vi "PNA_yokogawa_anritsu_combined.vi"() -> ()   [LabVIEW 2020]
uses:
  <vilib>/Utility/file.llb/Write Delimited Spreadsheet (DBL).vi
  <instrlib>/Keysight PNA Series/Keysight PNA Series.lvlib
  <instrlib>/Anritsu MG369X Series/Anritsu MG369X Series.lvlib
  <instrlib>/Yokogawa 7651/Yokogawa 7651.lvlib
panel:
  in  "Increment cluster":T1={"Yoko_Increment"=0.02, "Micro_Increment (GHz)"=0.1}
  in  "PNA_control":T2={"Channel (1)"=1, "Start Frequency (Hz)"=1000000.0, "Stop Frequency (Hz)"=10000000000.0, "Sweep Points (201)"=201, "Sweep Type (0: Linear)"=0, "Sweep Generation (1: Analog)"=1, "Bandwidth (Hz)"=100000.0, "Average Count (1)"=1, "Enable Average "=FALSE, "Power"={"Attenuation (0 dB)"=0.0, "Power Level (0 dBm)"=0.0, "Enable Auto Attenuation"=TRUE, "Enable RF Power"=TRUE, "Enable Power Slope"=FALSE, "Port (1)"=1, "Power Slope (0 dB/GHz)"=0.0}, "Enable Reduce IF Bandwidth "=TRUE, "Electrical delay"={"Unit (0: Meter)"=0, "Waveguide Cutoff Frequency (Hz)"=45000000.0, "Distance (0)"=0.0, "Medium "=0, "Delay (0 s)"=0.0}, "Measurement name"=[], "Measurement Parameters (S11)"=[]} {"Electrical delay"."Medium" items=["Coaxial", "Waveguide"]; "Electrical delay"."Unit (0: Meter)" items=["Meter", "Feet", "Inch"]; "Sweep Generation (1: Analog)" items=["Stepped", "Analog"]; "Sweep Type (0: Linear)" items=["Linear", "Logarithmic", "Power", "CW", "Segment", "Phase"]}
  in  "VNA_force_stop":bool
  in  "Save?":bool
  in  "Save file path":path=path "D:/Sheng-Xiang_Lin/JPA"
  in  "File_name":string="JPA"
  in  "Yoko_control":T3={"Range"=enum."10mA", "Init_Current/ Voltage "=1.46}
  in  "Output_control":T4
  in  "MicroScan_or_YokoScan":enum16{"MicroScan", "YokoScan"}(ring)=enum."YokoScan"
  in  "Display format 1-2":T5={"Display Format 2"=3, "Display Format 1"=1} {"Display Format 1" items=["Magnitude Linear", "Magnitude Logarithmic", "Phase", "Unwrapped phase", "Imaginary", "Real", "Polar", "Smith Chart", "Smith Admittance", "SWR", "Group Delay", "Kelvin", "Fahrenheit", "Celsius"]; "Display Format 2" items=["Magnitude Linear", "Magnitude Logarithmic", "Phase", "Unwrapped phase", "Imaginary", "Real", "Polar", "Smith Chart", "Smith Admittance", "SWR", "Group Delay", "Kelvin", "Fahrenheit", "Celsius"]}
  out "average_times":i32=1
  in  "MG369X_control":T6={"Initial Frequency (Hz)"=4000000000.0, "Initial Power Level (dBm)"=0.0, "Trigger Type (1: Free Run)"=1, "Clock Rate (4: Clock 100)"=1, "Trigger Edge Type (0: Trigger Rising)"=0, "Polarity (1: High RF On)"=1, "Pulse_Period (s)"=1e-08, "Mode (1: Single)"=1, "Reset (True)"=FALSE, "ID Query (True)"=FALSE} {"Mode (1: Single)" items=["Single"=1, "Doublet"=2, "Triplet"=3, "Quadruplet"=4]; "Pulse_Period (s)" format="%#_12g"; "Polarity (1: High RF On)" items=["Low RF On", "High RF On"]; "Trigger Edge Type (0: Trigger Rising)" items=["Trigger Rising", "Trigger Falling"]; "Clock Rate (4: Clock 100)" items=["Clock 10"=1, "Clock 100"=4]; "Trigger Type (1: Free Run)" items=["Free Run"=1, "Gated"=2, "Delayed"=3, "Triggered"=4, "Triggered w/delay"=5]}
  in  "Force_stop":bool
  out "State":T7(ring)=enum."Close"
  in  "Limit_Cluster":T8={"Current_or_voltage_limit"=1.5, "Micro_freq_limit (GHz)"=4.5}
  in  "Current_Value":T9={"Yoko_Current_or_Voltage"=1.52, "Micro_frequency (GHz)"=4.0, "Ch1 Intensity Graph"=array2001x3[6003 elements], "Freq_Array"=array[2001 elements], "Ch2 Intensity Graph"=array2001x3[6003 elements], "Ch1"={"Magnitude"=array[201 elements], "Phase"=array[201 elements]}, "Ch2"={"Magnitude"=array[201 elements], "Phase"=array[201 elements]}}
  in  "Leave_pend":bool
  in  "Visa_Cluster":T10={"VNA visa"="GPIB0::16::INSTR", "MG369x visa"="GPIB0::5::INSTR", "Yokogawa visa"="GPIB0::1::INSTR"}
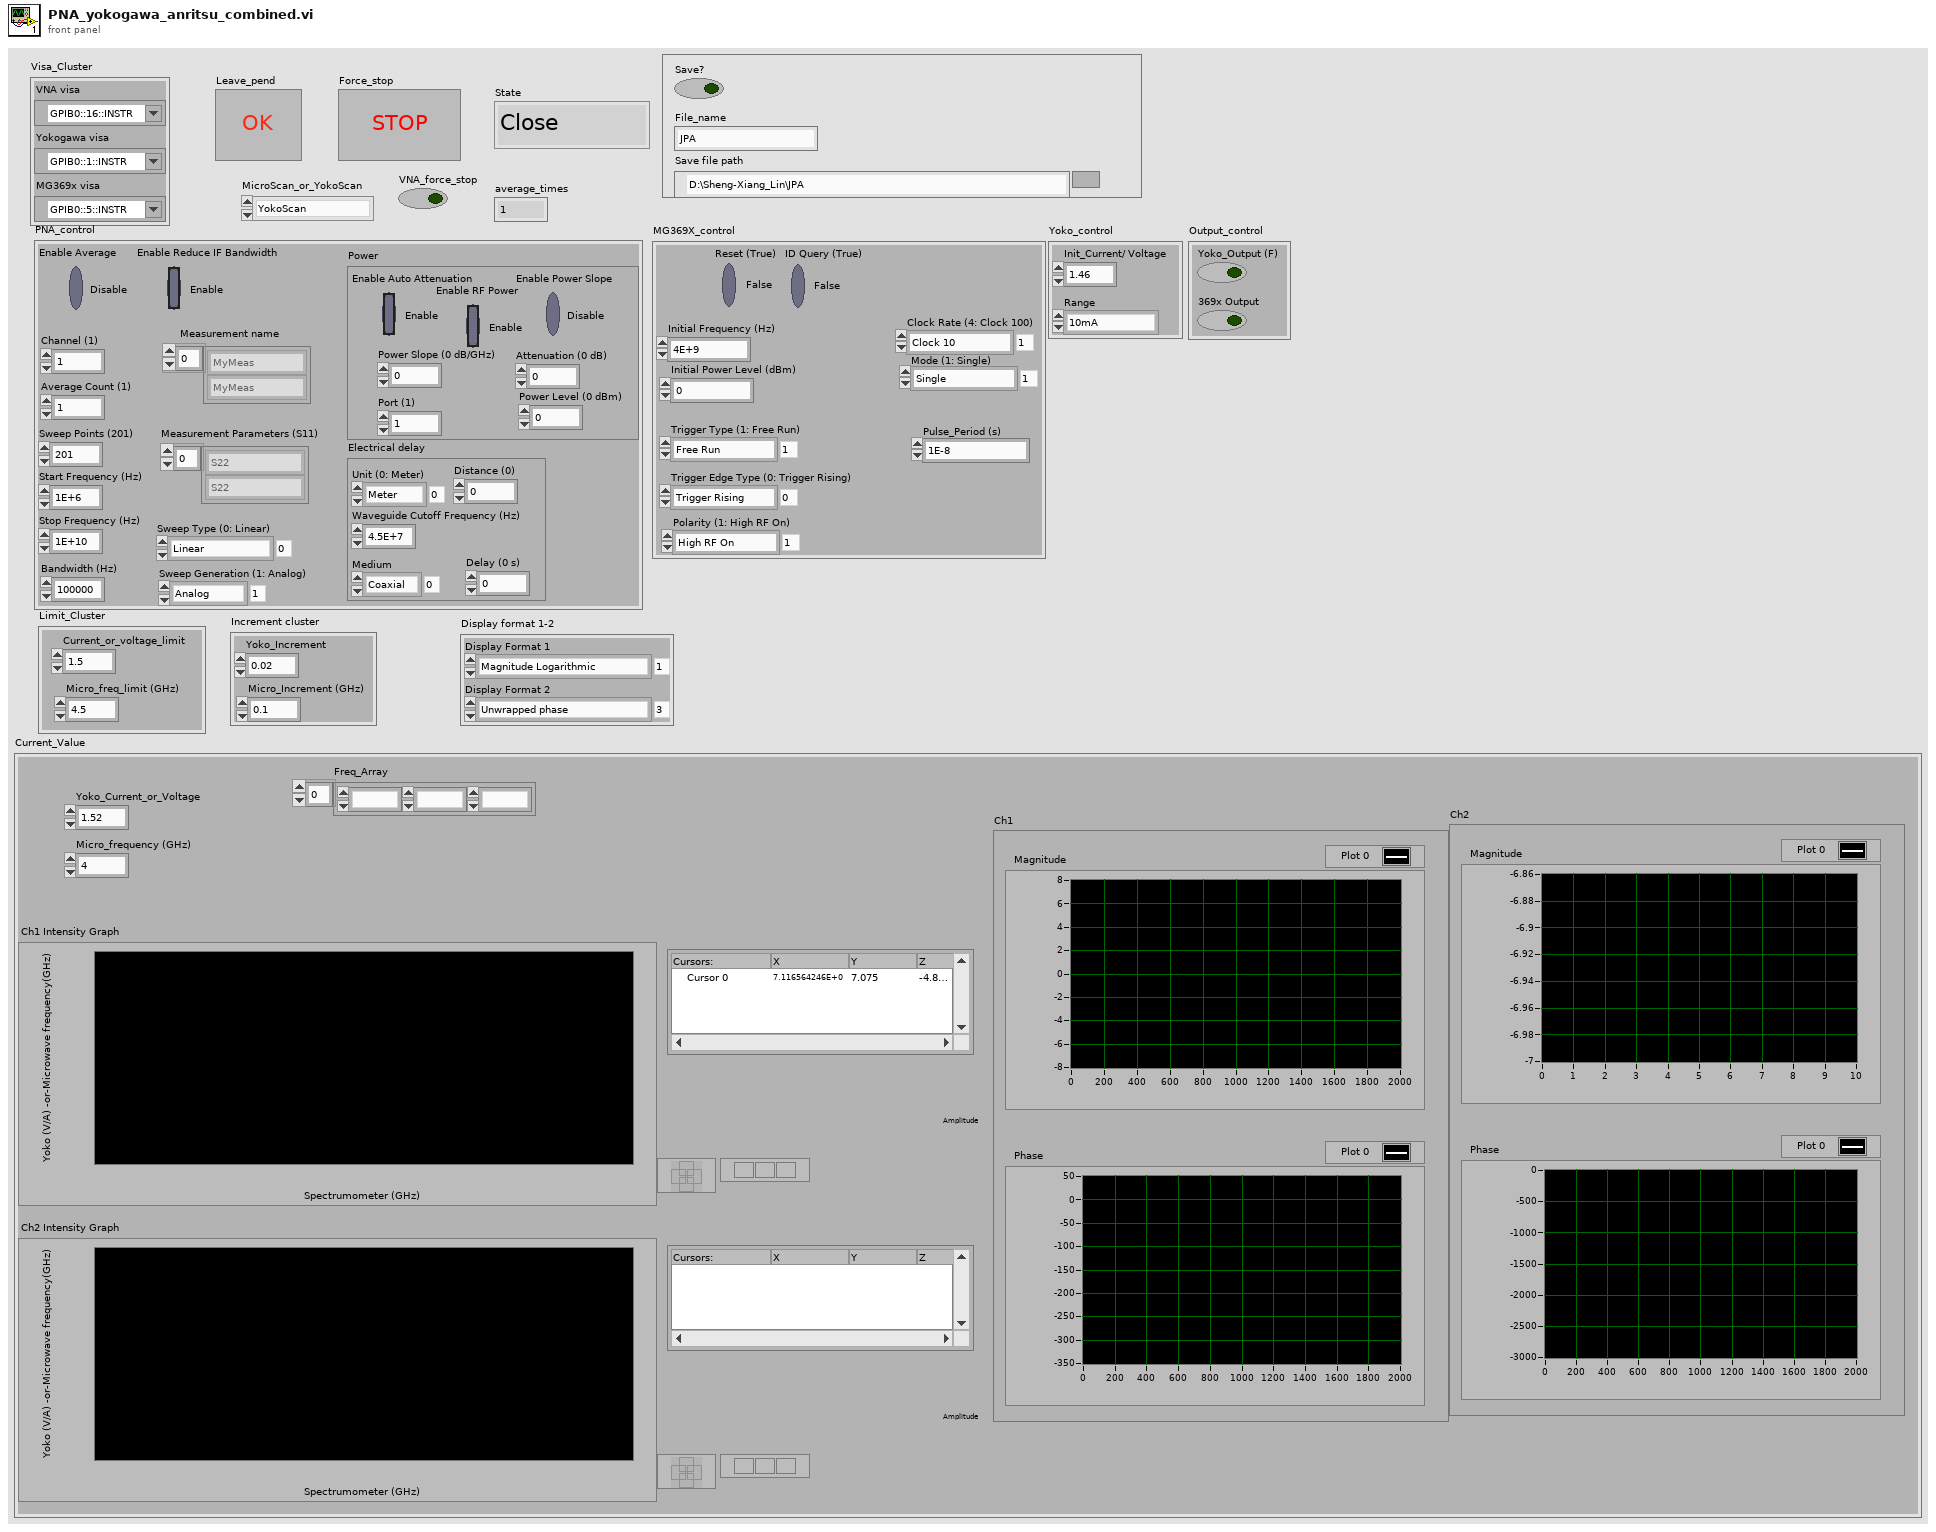
[diagram p1: front panel]
types:
  T1 = cluster{"Yoko_Increment":dbl, "Micro_Increment (GHz)":dbl}
  T2 = cluster{"Channel (1)":i32, "Start Frequency (Hz)":dbl, "Stop Frequency (Hz)":dbl, "Sweep Points (201)":i32, "Sweep Type (0: Linear)":i32, "Sweep Generation (1: Analog)":i32, "Bandwidth (Hz)":dbl, "Average Count (1)":i32, "Enable Average ":bool, "Power":cluster{"Attenuation (0 dB)":dbl, "Power Level (0 dBm)":dbl, "Enable Auto Attenuation":bool, "Enable RF Power":bool, "Enable Power Slope":bool, "Port (1)":i32, "Power Slope (0 dB/GHz)":dbl}, "Enable Reduce IF Bandwidth ":bool, "Electrical delay":cluster{"Unit (0: Meter)":i32, "Waveguide Cutoff Frequency (Hz)":dbl, "Distance (0)":dbl, "Medium ":i32, "Delay (0 s)":dbl}, "Measurement name":string[], "Measurement Parameters (S11)":string[]}
  T3 = cluster{"Range":enum16{"10mV", "100mV", "1V", "10V", "30V", "1mA", "10mA", "100mA"}, "Init_Current/ Voltage ":dbl}
  T4 = cluster{"Yoko_Output (F)":bool, "369x Output":bool}
  T5 = cluster{"Display Format 2":i32, "Display Format 1":i32}
  T6 = cluster{"Initial Frequency (Hz)":dbl, "Initial Power Level (dBm)":dbl, "Trigger Type (1: Free Run)":u16, "Clock Rate (4: Clock 100)":u16, "Trigger Edge Type (0: Trigger Rising)":u16, "Polarity (1: High RF On)":u16, "Pulse_Period (s)":dbl, "Mode (1: Single)":u16, "Reset (True)":bool, "ID Query (True)":bool}
  T7 = enum16{"Init", "Pend", "micro_scan", "Yogo_scan", "VNA_result", "Close", "Save_and_write", "VNA_configure"}
  T8 = cluster{"Current_or_voltage_limit":dbl, "Micro_freq_limit (GHz)":dbl}
  T9 = cluster{"Yoko_Current_or_Voltage":dbl, "Micro_frequency (GHz)":dbl, "Ch1 Intensity Graph":dbl[][], "Freq_Array":dbl[], "Ch2 Intensity Graph":dbl[][], "Ch1":cluster{"Magnitude":dbl[], "Phase":dbl[]}, "Ch2":cluster{"Magnitude":dbl[], "Phase":dbl[]}}
  T10 = cluster{"VNA visa":refnum<visa-resource-name>, "MG369x visa":refnum<visa-resource-name>, "Yokogawa visa":refnum<visa-resource-name>}
  T11 = enum16{"Init", "Pend", "micro_scan", "Yogo_scan", "VNA_result", "Close"}
  T12 = enum16{"Init", "Pend", "micro_scan", "Yogo_scan", "VNA_result", "Close", "Save_and_write"}
  T13 = enum16{"10mV", "100mV", "1V", "10V", "30V", "1mA", "10mA", "100mA"}
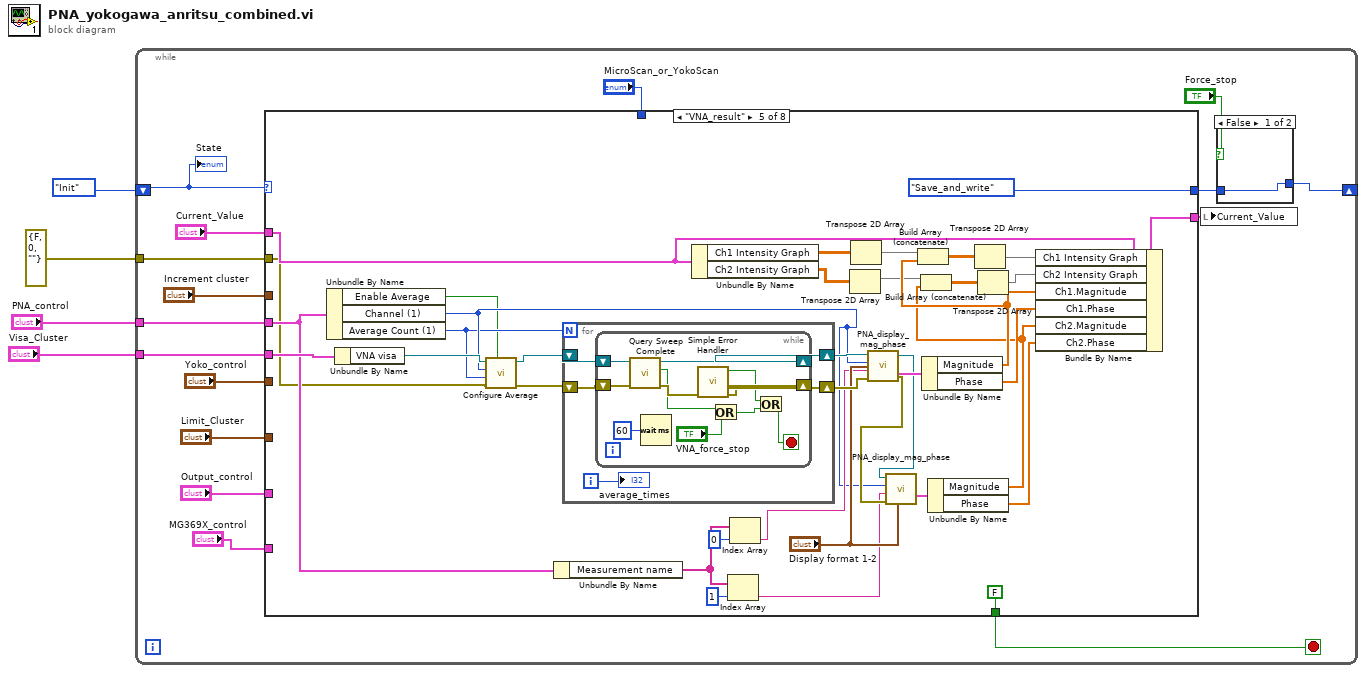
[diagram p0: block diagram]
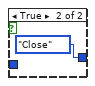
[diagram p2: hidden frame]
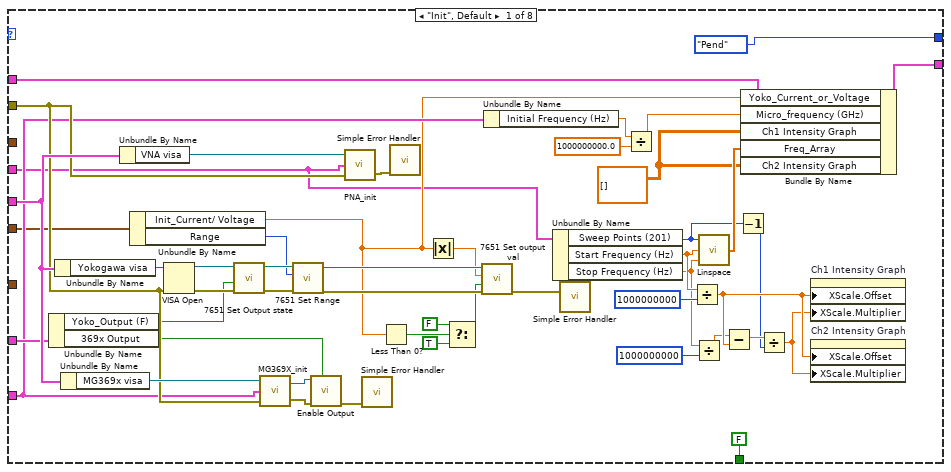
[diagram p3: hidden frame]
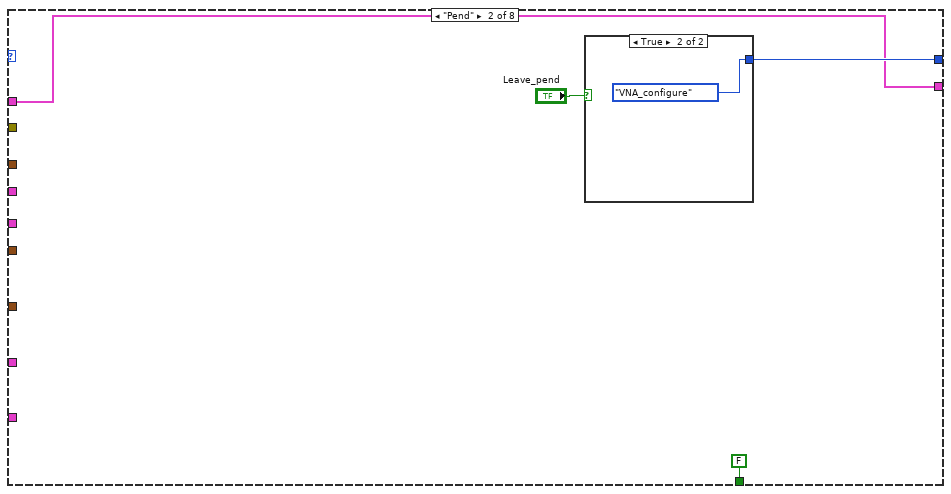
[diagram p4: hidden frame]
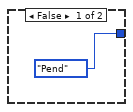
[diagram p5: hidden frame]
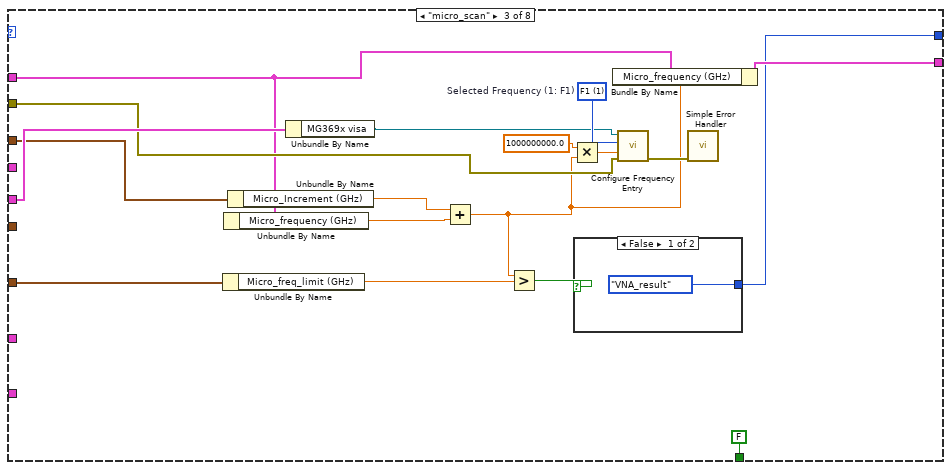
[diagram p6: hidden frame]
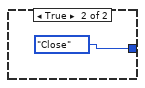
[diagram p7: hidden frame]
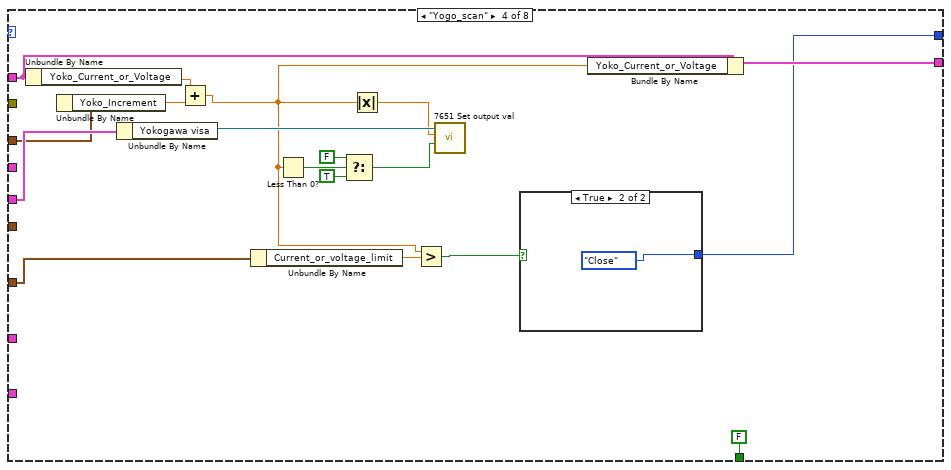
[diagram p8: hidden frame]
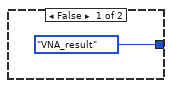
[diagram p9: hidden frame]
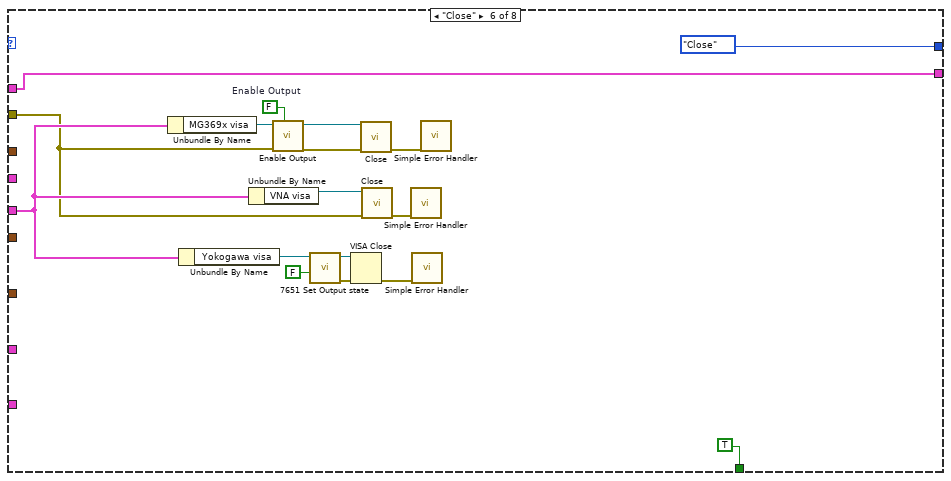
[diagram p10: hidden frame]
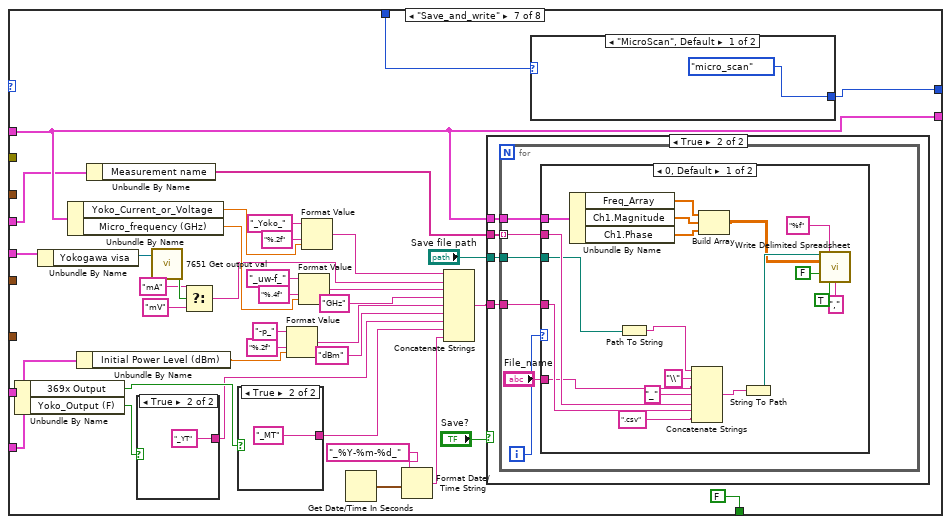
[diagram p11: hidden frame]
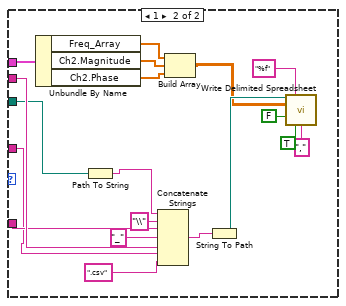
[diagram p13: hidden frame]
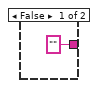
[diagram p14: hidden frame]
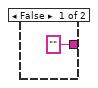
[diagram p15: hidden frame]
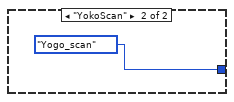
[diagram p16: hidden frame]
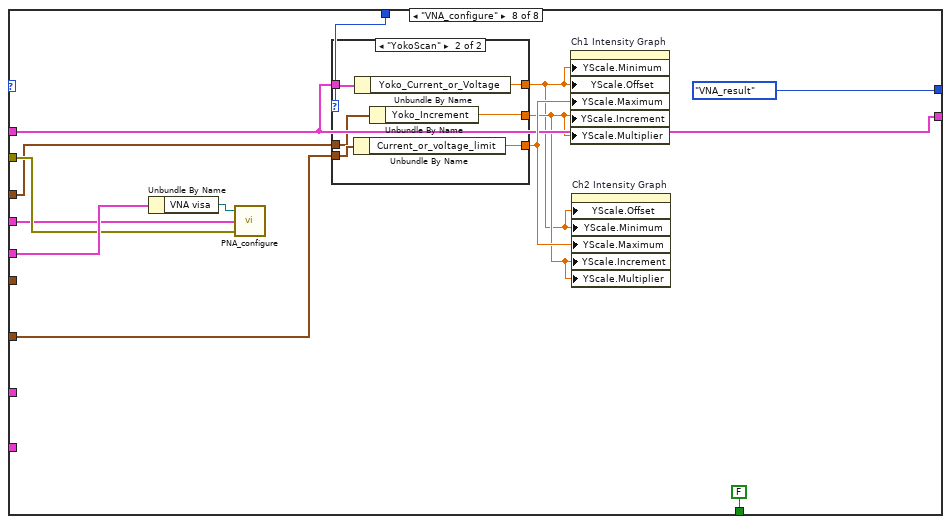
[diagram p17: hidden frame]
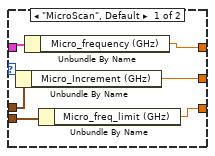
[diagram p18: hidden frame]
diagram:
  n1 = while {
    tunnel: errorcluster {"status"=FALSE, "code"=0, "source"=""} ("error in (no error)") -> [w20]
    tunnel: "Visa_Cluster" -> [w19]
    shift-right: [w14] -> _
    shift-left: T7."Init" ("State 2") -> [w7]
    tunnel: "PNA_control" -> [w8]
    stop <- w12 stop-if-true
    n2 = case shown="\"VNA_result\"" w7 {
      tunnel: w20 -> [w55 _ w91 _ w121 w174 _ w289]
      tunnel: w19 -> [w58 _ w93 w110 w153 w176 w213 w291]
      tunnel: [T11."Pend" ("State") w74 w84 w101 T12."Save_and_write" ("State") T11."Close" ("State") w224 T7."VNA_result" ("State 2")] -> w13
      tunnel: [w52 w71 w90 w106 w143 w172 w194 w283] -> w18
      tunnel: "Current_Value" -> [w53 w71 w89 w107 w151 w172 w194 w283]
      tunnel: "Limit_Cluster" -> [_ _ w87 w102 _ _ _ w282]
      tunnel: [FALSE FALSE FALSE FALSE FALSE TRUE FALSE FALSE] -> w12
      tunnel: "Output_control" -> [w41 _ _ _ _ _ w202 _]
      tunnel: "MG369X_control" -> [w38 _ _ _ _ _ w215 _]
      tunnel: "Yoko_control" -> [w37 _ _ _ _ _ _ _]
      tunnel: w8 -> [w34 _ _ _ w124 _ w193 w288]
      tunnel: "MicroScan_or_YokoScan" -> [_ _ _ _ _ _ w187 w284]
      tunnel: "Increment cluster" -> [_ _ w78 w97 _ _ _ w281]
      frame "Init", Default {
        w33 = dbl[][] [] ("Intensity Graph")
        n3 = Unbundle By Name(w41) -> ("Yoko_Output (F)"=w40:bool, "369x Output"=w39:bool)
        n4 = Unbundle By Name(w58) -> ("Yokogawa visa"=w59:refnum<visa-resource-name>)
        n5 = Unbundle By Name(w58) -> ("MG369x visa"=w57:refnum<visa-resource-name>)
        n6 = Unbundle By Name(w58) -> ("VNA visa"=w56:refnum<visa-resource-name>)
        n7 = Unbundle By Name(w37) -> ("Init_Current/ Voltage"=w35:dbl, "Range"=w36:T13)
        n8 = VISA Open(error in (no error)=w55, VISA resource name=w59) -> (VISA resource name=w69:refnum<visa-resource-name>, error out=w70:errorcluster)  [unwired: 3 in]
        n9 = call <instrlib>:"7651 Set Output state.vi"("error in"=w70, "Output (F)"=w40, "VISA  name"=w69) -> ("error out"=w67:errorcluster, "VISA  name"=w66:refnum<visa-resource-name>)  [unwired: 7 in]
        n10 = call "MG369X_init.vi"("error in (no error)"=w55, "MG369X_control"=w38, "MG369X_VISA"=w57) -> ("error out"=w44:errorcluster, "MG369X_Visa_out"=w45:refnum<visa-resource-name>)
        n11 = call <instrlib>:"7651 Set Range.vi"("error in"=w67, "Range"=w36, "VISA  name"=w66) -> ("error out"=w68:errorcluster, "VISA  name"=w65:refnum<visa-resource-name>)  [unwired: 7 in]
        n12 = call <instrlib>:"Enable Output.vi"("Enable Output (F: Disable)"=w39, "error in (no error)"=w44, "VISA resource name"=w45) -> ("error out"=w43:errorcluster)  [unwired: 7 in, 1 out]
        n13 = call "PNA_init.vi"("error in (no error)"=w55, "PNA_control"=w34, "PNA_visa"=w56) -> ("error out"=w47:errorcluster)  [unwired: 1 out]
        n14 = call <vilib>:"Simple Error Handler.vi"("error in (no error)"=w43) -> ()  [unwired: 4 in, 5 out]
        n15 = Less Than 0?(x=w35) -> (x < 0?=w64:bool)
        n16 = call <vilib>:"Simple Error Handler.vi"("error in (no error)"=w47) -> ()  [unwired: 4 in, 5 out]
        n17 = Absolute Value(x=w35) -> (abs(x)=w60:dbl)
        n18 = Select(t=FALSE, s=w64, f=TRUE) -> (s? t:f=w61:bool)
        n19 = call <instrlib>:"7651 Set output val.vi"("error in"=w68, "Pol (T)"=w61, "Val mV/mA (0)"=w60, "VISA  name"=w65) -> ("error out"=w46:errorcluster)  [unwired: 6 in, 1 out]
        n20 = Unbundle By Name(w38) -> ("Initial Frequency (Hz)"=w49:dbl)
        n21 = Unbundle By Name(w34) -> ("Sweep Points (201)"=w23:i32, "Start Frequency (Hz)"=w32:dbl, "Stop Frequency (Hz)"=w29:dbl)
        n22 = call <vilib>:"Simple Error Handler.vi"("error in (no error)"=w46) -> ()  [unwired: 4 in, 5 out]
        n23 = Divide(x=w49, y=1000000000.0) -> (x/y=w48:dbl)
        n24 = Divide(x=w32, y=i64 1000000000) -> (x/y=w28:dbl)
        n25 = Divide(x=w29, y=i64 1000000000) -> (x/y=w27:dbl)
        n26 = call "Linspace.vi"("Stop_value"=w29, "Start_value"=w32, "Num"=w23) -> ("Output_array"=w42:dbl[])
        n27 = Subtract(x=w27, y=w28) -> (x-y=w26:dbl)
        n28 = Decrement(x=w23) -> (x-1=w24:i32)
        n29 = Bundle By Name(cluster=w53, "Yoko_Current_or_Voltage"=w35, "Micro_frequency (GHz)"=w48, "Ch1 Intensity Graph"=w33, "Freq_Array"=w42, "Ch2 Intensity Graph"=w33) -> (w52:T9)
        n30 = Divide(x=w26, y=w24) -> (x/y=w25:dbl)
        n31 = property on="Ch1 Intensity Graph" class="IntGraph (strict)"("XScale.Offset"=w28, "XScale.Multiplier"=w25) -> ()  [unwired: 2 in, 2 out]
        n32 = property on="Ch2 Intensity Graph" class="IntGraph (strict)"("XScale.Offset"=w28, "XScale.Multiplier"=w25) -> ()  [unwired: 2 in, 2 out]
      }
      frame "Pend" {
        n33 = case shown="True" "Leave_pend" {
          tunnel: [T7."Pend" ("State 2") T7."VNA_configure" ("State 2")] -> w74
          frame False {
          }
          frame True {
          }
        }
      }
      frame "micro_scan" {
        w94 = u16 1 items=["F0", "F1", "F2", "F3", "F4", "F5", "F6", "F7", "F8", "F9", "M0", "M1", "M2", "M3", "M4", "M5", "M6", "M7", "M8", "M9"]  # Selected Frequency (1: F1)
        n34 = Unbundle By Name(w87) -> ("Micro_freq_limit (GHz)"=w86:dbl)
        n35 = Unbundle By Name(w89) -> ("Micro_frequency (GHz)"=w88:dbl)
        n36 = Unbundle By Name(w78) -> ("Micro_Increment (GHz)"=w77:dbl)
        n37 = Unbundle By Name(w93) -> ("MG369x visa"=w92:refnum<visa-resource-name>)
        n38 = Add(x=w77, y=w88) -> (x+y=w79:dbl)
        n39 = Greater?(x=w79, y=w86) -> (0:w85:bool)
        n40 = Multiply(x=1000000000.0 ("y"), y=w79) -> (x*y=w81:dbl)
        n41 = case shown="False" w85 {
          tunnel: [T11."VNA_result" ("State") T11."Close" ("State")] -> w84
          frame False {
          }
          frame True {
          }
        }
        n42 = Bundle By Name(cluster=w89, "Micro_frequency (GHz)"=w79) -> (w90:T9)
        n43 = call <instrlib>:"Configure Frequency Entry.vi"("error in (no error)"=w91, "Frequency (2.2E+9 Hz)"=w81, "Selected Frequency (1: F1)"=w94, "VISA resource name"=w92) -> ("error out"=w82:errorcluster)  [unwired: 6 in, 1 out]
        n44 = call <vilib>:"Simple Error Handler.vi"("error in (no error)"=w82) -> ()  [unwired: 4 in, 5 out]
      }
      frame "Yogo_scan" {
        n45 = Unbundle By Name(w107) -> ("Yoko_Current_or_Voltage"=w108:dbl)
        n46 = Unbundle By Name(w97) -> ("Yoko_Increment"=w98:dbl)
        n47 = Unbundle By Name(w110) -> ("Yokogawa visa"=w109:refnum<visa-resource-name>)
        n48 = Add(x=w108, y=w98) -> (x+y=w99:dbl)
        n49 = Unbundle By Name(w102) -> ("Current_or_voltage_limit"=w103:dbl)
        n50 = Less Than 0?(x=w99) -> (x < 0?=w114:bool)
        n51 = Select(t=FALSE, s=w114, f=TRUE) -> (s? t:f=w111:bool)
        n52 = Absolute Value(x=w99) -> (abs(x)=w105:dbl)
        n53 = Greater?(x=w99, y=w103) -> (0:w104:bool)
        n54 = call <instrlib>:"7651 Set output val.vi"("Pol (T)"=w111, "Val mV/mA (0)"=w105, "VISA  name"=w109) -> ()  [unwired: 7 in, 2 out]
        n55 = case shown="True" w104 {
          tunnel: [T11."VNA_result" ("State") T11."Close" ("State")] -> w101
          frame False {
          }
          frame True {
          }
        }
        n56 = Bundle By Name(cluster=w107, "Yoko_Current_or_Voltage"=w99) -> (w106:T9)
      }
      frame "VNA_result" {
        n57 = Unbundle By Name(w124) -> ("Enable Average"=w117:bool, "Channel (1)"=w119:i32, "Average Count (1)"=w118:i32)
        n58 = Unbundle By Name(w153) -> ("VNA visa"=w120:refnum<visa-resource-name>)
        n59 = call <instrlib>:"Configure Average.vi"("Enable Average (F: Disable)"=w117, "error in (no error)"=w121, "Average Count (1)"=w118, "Channel (1)"=w119, "VISA resource name"=w120) -> ("error out"=w122:errorcluster, "VISA resource name out"=w123:refnum<visa-resource-name>)  [unwired: 5 in]
        n60 = Unbundle By Name(w124) -> ("Measurement name"=w129:string[])
        n61 = for {
          N: w118 -> [_]
          shift-right: [w158] -> w147
          shift-left: w123 -> [w155]
          shift-right: [w157] -> w146
          shift-left: w122 -> [w154]
          i -> [w156]
          n62 = while {
            shift-right: [w164] -> w157
            shift-left: w154 -> [w169]
            shift-right: [w167] -> w158
            shift-left: w155 -> [w168]
            stop <- w162 stop-if-true
            n63 = call <instrlib>:"Query Sweep Complete.vi"("error in (no error)"=w169, "VISA resource name"=w168) -> ("error out"=w165:errorcluster, "Sweep Complete"=w160:bool, "VISA resource name out"=w167:refnum<visa-resource-name>)  [unwired: 7 in]
            n64 = Wait (ms)(milliseconds to wait=u32 60) -> ()  [unwired: 1 out]
            n65 = call <vilib>:"Simple Error Handler.vi"("error in (no error)"=w165) -> ("error?"=w163:bool, "error out"=w164:errorcluster)  [unwired: 4 in, 3 out]
            n66 = Or(x=w160, y="VNA_force_stop") -> (x .or. y?=w161:bool)
            n67 = Or(x=w163, y=w161) -> (x .or. y?=w162:bool)
          }
          "average_times" <- w156
        }
        n68 = Unbundle By Name(w151) -> ("Ch1 Intensity Graph"=w150:dbl[][], "Ch2 Intensity Graph"=w135:dbl[][])
        n69 = Index Array(array=w129, index=1) -> (element=w125:string)
        n70 = Index Array(array=w129, index=0) -> (element=w126:string)
        n71 = Transpose 2D Array(2D array=w135) -> (transposed array=w132:dbl[][])
        n72 = Transpose 2D Array(2D array=w150) -> (transposed array=w149:dbl[][])
        n73 = call "PNA_display_mag_phase.vi"("VISA resource name"=w147, "Channel (1)"=w119, "Measurement Name (CH1_S11)"=w126, "error in (no error)"=w146, "Display format 1-2"="Display format 1-2") -> ("VISA resource name out"=w140:refnum<visa-resource-name>, "Cluster"=w145:cluster{"Magnitude":dbl[], "Phase":dbl[]}, "error out"=w139:errorcluster)
        n74 = call "PNA_display_mag_phase.vi"("VISA resource name"=w140, "Channel (1)"=w119, "Measurement Name (CH1_S11)"=w125, "error in (no error)"=w139, "Display format 1-2"="Display format 1-2") -> ("Cluster"=w137:cluster{"Magnitude":dbl[], "Phase":dbl[]})  [unwired: 2 out]
        n75 = Unbundle By Name(w145) -> ("Magnitude"=w142:dbl[], "Phase"=w141:dbl[])
        n76 = Build Array (concatenate)(w149, w142) -> (w148:dbl[][])
        n77 = Unbundle By Name(w137) -> ("Magnitude"=w130:dbl[], "Phase"=w136:dbl[])
        n78 = Build Array (concatenate)(w132, w130) -> (w133:dbl[][])
        n79 = Transpose 2D Array(2D array=w148) -> (transposed array=w134:dbl[][])
        n80 = Transpose 2D Array(2D array=w133) -> (transposed array=w131:dbl[][])
        n81 = Bundle By Name(cluster=w151, "Ch1 Intensity Graph"=w134, "Ch2 Intensity Graph"=w131, "Ch1.Magnitude"=w142, "Ch1.Phase"=w141, "Ch2.Magnitude"=w130, "Ch2.Phase"=w136) -> (w143:T9)
      }
      frame "Close" {
        w179 = FALSE  # Enable Output
        n82 = Unbundle By Name(w176) -> ("MG369x visa"=w175:refnum<visa-resource-name>)
        n83 = Unbundle By Name(w176) -> ("Yokogawa visa"=w180:refnum<visa-resource-name>)
        n84 = Unbundle By Name(w176) -> ("VNA visa"=w185:refnum<visa-resource-name>)
        n85 = call <instrlib>:"Enable Output.vi"("Enable Output (F: Disable)"=w179, "error in (no error)"=w174, "VISA resource name"=w175) -> ("error out"=w177:errorcluster, "VISA resource name out"=w178:refnum<visa-resource-name>)  [unwired: 7 in]
        n86 = call <instrlib>:"7651 Set Output state.vi"("Output (F)"=FALSE, "VISA  name"=w180) -> ("error out"=w184:errorcluster, "VISA  name"=w183:refnum<visa-resource-name>)  [unwired: 8 in]
        n87 = VISA Close(VISA resource name=w183, error in (no error)=w184) -> (error out=w181:errorcluster)
        n88 = call <instrlib>:"Close.vi"("error in (no error)"=w177, "VISA resource name"=w178) -> ("error out"=w173:errorcluster)  [unwired: 9 in]
        n89 = call <instrlib>:"Close.vi"("error in (no error)"=w174, "VISA resource name"=w185) -> ("error out"=w186:errorcluster)  [unwired: 9 in]
        n90 = call <vilib>:"Simple Error Handler.vi"("error in (no error)"=w186) -> ()  [unwired: 4 in, 5 out]
        n91 = call <vilib>:"Simple Error Handler.vi"("error in (no error)"=w181) -> ()  [unwired: 4 in, 5 out]
        n92 = call <vilib>:"Simple Error Handler.vi"("error in (no error)"=w173) -> ()  [unwired: 4 in, 5 out]
      }
      frame "Save_and_write" {
        n93 = Unbundle By Name(w202) -> ("369x Output"=w200:bool, "Yoko_Output (F)"=w201:bool)
        n94 = Unbundle By Name(w213) -> ("Yokogawa visa"=w212:refnum<visa-resource-name>)
        n95 = Unbundle By Name(w194) -> ("Yoko_Current_or_Voltage"=w221:dbl, "Micro_frequency (GHz)"=w218:dbl)
        n96 = Unbundle By Name(w215) -> ("Initial Power Level (dBm)"=w214:dbl)
        n97 = Unbundle By Name(w193) -> ("Measurement name"=w192:string[])
        n98 = case shown="True" w201 {
          tunnel: ["" "_YT"] -> w199
          frame False {
          }
          frame True {
          }
        }
        n99 = call <instrlib>:"7651 Get output val.vi"("VISA  name"=w212) -> ("mV / mA (T=mA)"=w211:bool)  [unwired: 4 in, 6 out]
        n100 = Select(t="mA" ("string (\"\")"), s=w211, f="mV") -> (s? t:f=w207:string)
        n101 = case shown="True" w200 {
          tunnel: ["" "_MT"] -> w198
          frame False {
          }
          frame True {
          }
        }
        n102 = Format Value(string ("")="-p_", format string="%.2f", value (0)=w214) -> (output string=w204:string)
        n103 = Format Value(string ("")="_uw-f_", format string="%.4f", value (0)=w218) -> (output string=w206:string)
        n104 = Format Value(string ("")="_Yoko_", format string="%.2f", value (0)=w221) -> (output string=w208:string)
        n105 = Get Date/Time In Seconds() -> (seconds since 1Jan1904=w197:timestamp)
        n106 = Format Date/Time String(time format string (%c)="_%Y-%m-%d_", seconds (now)=w197) -> (date/time string=w195:string)  [unwired: 1 in]
        n107 = Concatenate Strings(w208, w207, w206, "GHz" ("string (\"\")"), w204, "dBm" ("string"), w199, w198, w195) -> (w191:string)
        n108 = case shown="True" "Save?" {
          tunnel: w194 -> [_ w228]
          tunnel: w192 -> [_ w227]
          tunnel: w191 -> [_ w226]
          tunnel: "Save file path" -> [_ w225]
          frame False {
          }
          frame True {
            n109 = for {
              tunnel: w228 -> [w233]
              tunnel: w227 -> [w232] mode=indexing
              tunnel: w226 -> [w231]
              tunnel: w225 -> [w230]
              i -> [w234]
              n110 = case shown="0, Default" w234 {
                tunnel: w233 -> [w239 w258]
                tunnel: w232 -> [w238 w257]
                tunnel: w231 -> [w237 w254]
                tunnel: w230 -> [w236 w256]
                tunnel: "File_name" -> [w235 w255]
                frame 0, Default {
                  n111 = Unbundle By Name(w239) -> ("Freq_Array"=w245:dbl[], "Ch1.Magnitude"=w243:dbl[], "Ch1.Phase"=w244:dbl[])
                  n112 = Path To String(path=w236) -> (string=w240:string)
                  n113 = Concatenate Strings(w240, "\\" ("string"), w235, "_" ("input 2"), w238, w237, ".csv" ("input 3")) -> (w247:string)
                  n114 = Build Array(w245, w243, w244) -> (w242:dbl[][])
                  n115 = String To Path(string=w247) -> (path=w246:path)
                  n116 = call-poly <vilib>:"Write Delimited Spreadsheet.vi"("file path (dialog if empty)"=w246, "format (%.3f)"="%f", "2D data"=w242, "append to file? (new file:F)"=FALSE, "transpose? (no:F)"=TRUE, "delimiter (\\t)"="," ("delimiter (\\t)")) -> ()  [unwired: 8 in, 2 out]
                }
                frame 1 {
                  n117 = Unbundle By Name(w258) -> ("Freq_Array"=w264:dbl[], "Ch2.Magnitude"=w262:dbl[], "Ch2.Phase"=w263:dbl[])
                  n118 = Path To String(path=w256) -> (string=w259:string)
                  n119 = Concatenate Strings(w259, "\\" ("string"), w255, "_" ("input 2"), w257, w254, ".csv" ("input 3")) -> (w266:string)
                  n120 = Build Array(w264, w262, w263) -> (w261:dbl[][])
                  n121 = String To Path(string=w266) -> (path=w265:path)
                  n122 = call-poly <vilib>:"Write Delimited Spreadsheet.vi"("file path (dialog if empty)"=w265, "format (%.3f)"="%f", "2D data"=w261, "append to file? (new file:F)"=FALSE, "transpose? (no:F)"=TRUE, "delimiter (\\t)"="," ("delimiter (\\t)")) -> ()  [unwired: 8 in, 2 out]
                }
              }
            }
          }
        }
        n123 = case shown="\"MicroScan\", Default" w187 {
          tunnel: [T11."micro_scan" ("State") T11."Yogo_scan" ("State")] -> w224
          frame "MicroScan", Default {
          }
          frame "YokoScan" {
          }
        }
      }
      frame "VNA_configure" {
        n124 = Unbundle By Name(w291) -> ("VNA visa"=w290:refnum<visa-resource-name>)
        n125 = call "PNA_configure.vi"("error in (no error)"=w289, "PNA_control"=w288, "PNA_visa"=w290) -> ()  [unwired: 2 out]
        n126 = case shown="\"YokoScan\"" w284 {
          tunnel: w282 -> [w295 w301]
          tunnel: w283 -> [w297 w303]
          tunnel: [w296 w302] -> w279
          tunnel: [w294 w300] -> w285
          tunnel: w281 -> [w293 w299]
          tunnel: [w292 w298] -> w280
          frame "MicroScan", Default {
            n127 = Unbundle By Name(w293) -> ("Micro_Increment (GHz)"=w292:dbl)
            n128 = Unbundle By Name(w297) -> ("Micro_frequency (GHz)"=w296:dbl)
            n129 = Unbundle By Name(w295) -> ("Micro_freq_limit (GHz)"=w294:dbl)
          }
          frame "YokoScan" {
            n130 = Unbundle By Name(w301) -> ("Current_or_voltage_limit"=w300:dbl)
            n131 = Unbundle By Name(w303) -> ("Yoko_Current_or_Voltage"=w302:dbl)
            n132 = Unbundle By Name(w299) -> ("Yoko_Increment"=w298:dbl)
          }
        }
        n133 = property on="Ch1 Intensity Graph" class="IntGraph (strict)"("YScale.Minimum"=w279, "YScale.Offset"=w279, "YScale.Maximum"=w285, "YScale.Increment"=w280, "YScale.Multiplier"=w280) -> ()  [unwired: 2 in, 2 out]
        n134 = property on="Ch2 Intensity Graph" class="IntGraph (strict)"("YScale.Offset"=w279, "YScale.Minimum"=w279, "YScale.Maximum"=w285, "YScale.Increment"=w280, "YScale.Multiplier"=w280) -> ()  [unwired: 2 in, 2 out]
      }
    }
    n135 = local write "Current_Value"(w18) -> ()
    n136 = case shown="False" "Force_stop" {
      tunnel: [w21 T11."Close" ("State")] -> w14
      tunnel: w13 -> [w21 _]
      frame False {
      }
      frame True {
      }
    }
    "State" <- w7
  }
